vi "Processing the state after actuator action.vi"(8 "error in (no error)":errorcluster, 9 "Time to wait":i32=999, 10 "Actuator Name":string, 11 "UTP IO Session in":T1) -> (0 "error out":errorcluster, 1 "Error Text":string, 2 "Error code":i16, 3 "UTP IO Session out":T1, 4 "Result":i16, 5 "Error ocured?":bool, 7 "ExpiredTimeToWait?":bool)   [LabVIEW 2023, in "Actuators.lvlib"]
doc: "Processing the state after actuator action\nPeriod for reading is 10ms"
uses:
  Actuators.lvlib
  <vilib>/Noffz/UTP IO/UTP IO Library/Typedefs/Session Handle.ctl
  <vilib>/Noffz/UTP IO/UTP IO Library/UTP IO Pool Session.lvclass
  <vilib>/Noffz/UTP IO/UTP IO Library/methods/poly/plc/Read PLC Variable (Boolean).vi
  <vilib>/Noffz/UTP IO/UTP IO Library/methods/poly/plc/Read PLC Variable (I16).vi
  <vilib>/Noffz/UTP IO/UTP IO Library/methods/poly/plc/Read PLC Variable (String).vi
  <vilib>/Noffz/UTP IO/UTP IO Library/methods/poly/plc/Write PLC Variable (Boolean).vi
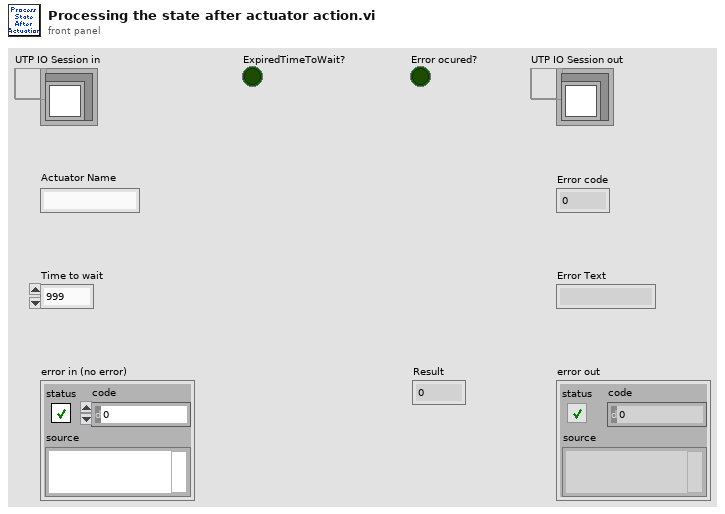
[diagram p1: front panel]
types:
  T1 = typedef "UTP IO Library.lvlib/UTP IO Pool Session.lvclass/Session Handle.ctl" = refnum<data-value>
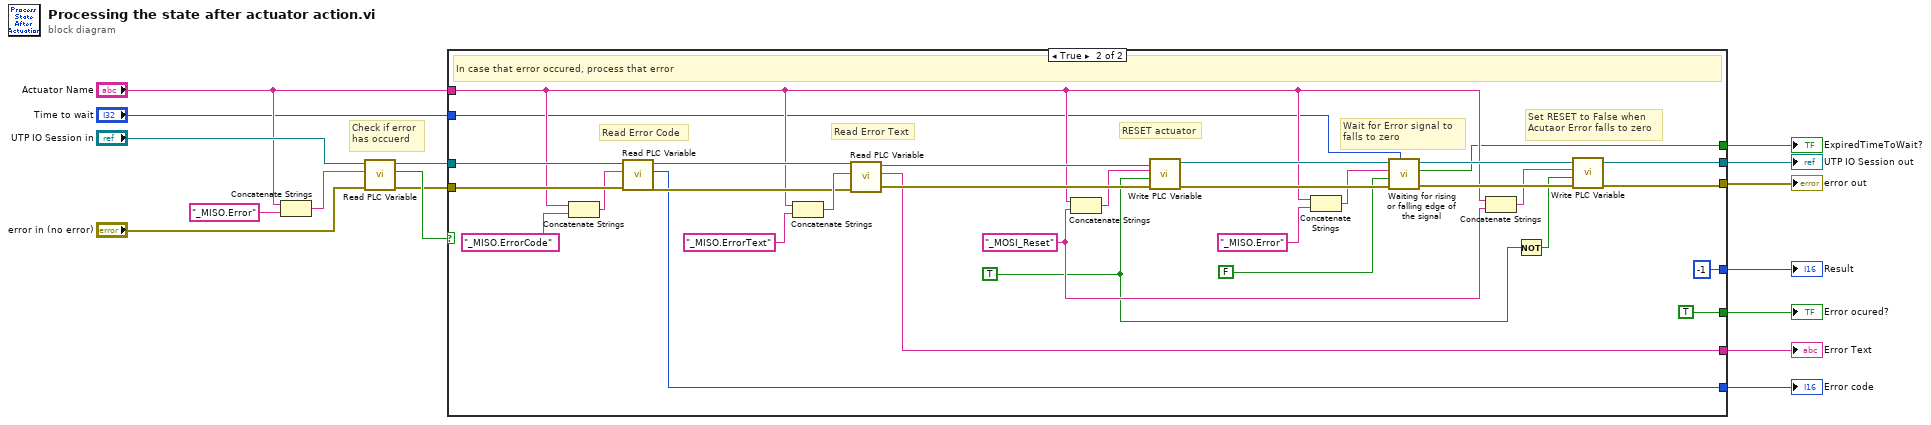
[diagram p0: block diagram]
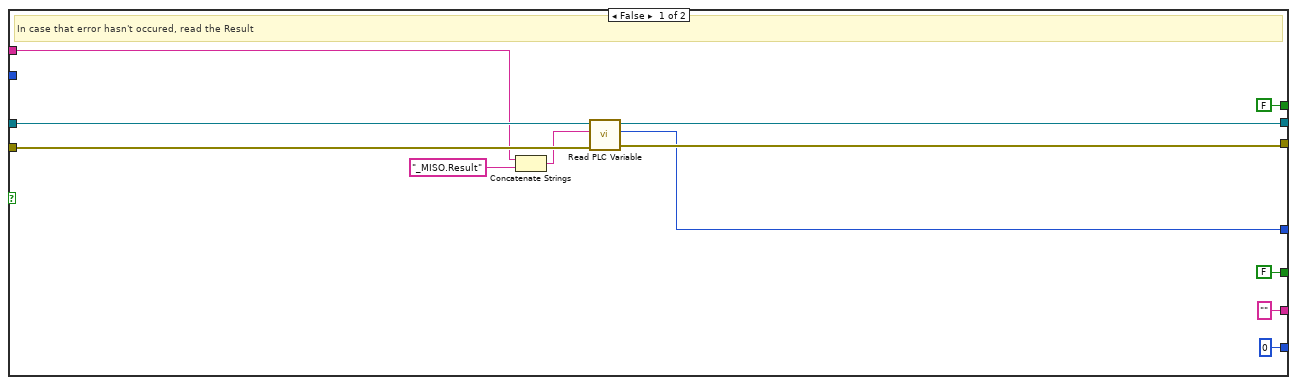
[diagram p2: hidden frame]
diagram:
  # "Check if error\nhas occuerd"
  n1 = Concatenate Strings("Actuator Name", "_MISO.Error" ("string")) -> (w14:string)
  n2 = call-poly <vilib>:"Read PLC Variable.vi"("error in (no error)"="error in (no error)", "variable name"=w14, "UTP IO Session in"="UTP IO Session in") -> ("error out"=w10:errorcluster, "value"=w15:bool, "UTP IO Session out"=w11:T1)  [unwired: 6 in]
  n3 = case shown="True" w15 {
    tunnel: w11 -> [w25 w59]
    tunnel: w10 -> [w23 w58]
    tunnel: "Actuator Name" -> [w19 w33]
    tunnel: [w24 w39] -> w3
    tunnel: [w22 w38] -> w8
    tunnel: ["" ("value") w37] -> w7
    tunnel: [i16 0 ("value") w36] -> w6
    tunnel: [FALSE ("Rising/Falling edge") TRUE ("Rising/Falling edge")] -> w5
    tunnel: [w18 i16 -1 ("value")] -> w4
    tunnel: [FALSE ("Expired3s?") w30] -> w2
    tunnel: "Time to wait" -> [_ w29]
    frame False {
      # "In case that error hasn't occured, read the Result"
      n4 = Concatenate Strings(w19, "_MISO.Result" ("string")) -> (w21:string)
      n5 = call-poly <vilib>:"Read PLC Variable.vi"("error in (no error)"=w23, "variable name"=w21, "UTP IO Session in"=w25) -> ("error out"=w22:errorcluster, "value"=w18:i16, "UTP IO Session out"=w24:T1)  [unwired: 6 in]
    }
    frame True {
      w40 = TRUE ("value")
      w43 = "_MOSI_Reset" ("string")
      # "Set RESET to False when\nAcutaor Error falls to zero"
      # "Wait for Error signal to \nfalls to zero"
      # "RESET actuator"
      # "Read Error Text"
      # "Read Error Code"
      # "In case that error occured, process that error"
      n6 = Concatenate Strings(w33, "_MISO.ErrorCode" ("string")) -> (w57:string)
      n7 = call-poly <vilib>:"Read PLC Variable.vi"("error in (no error)"=w58, "variable name"=w57, "UTP IO Session in"=w59) -> ("error out"=w52:errorcluster, "value"=w36:i16, "UTP IO Session out"=w56:T1)  [unwired: 6 in]
      n8 = Concatenate Strings(w33, "_MISO.ErrorText" ("string")) -> (w53:string)
      n9 = call-poly <vilib>:"Read PLC Variable.vi"("error in (no error)"=w52, "variable name"=w53, "UTP IO Session in"=w56) -> ("error out"=w50:errorcluster, "value"=w37:string, "UTP IO Session out"=w51:T1)  [unwired: 6 in]
      n10 = Concatenate Strings(w33, w43) -> (w49:string)
      n11 = call-poly <vilib>:"Write PLC Variable.vi"("error in (no error)"=w50, "value"=w40, "variable name"=w49, "UTP IO Session in"=w51) -> ("error out"=w47:errorcluster, "UTP IO Session out"=w48:T1)  [unwired: 6 in]
      n12 = Concatenate Strings(w33, "_MISO.Error" ("string")) -> (w31:string)
      n13 = call "Waiting for rising or falling edge of the signal.vi"("Time to wait"=w29, "error in"=w47, "Rising/Falling edge"=FALSE, "Variable name"=w31, "UTP IO Session in"=w48) -> ("error out"=w44:errorcluster, "ExpiredTimeToWait?"=w30:bool, "UTP IO Session out"=w45:T1)  [unwired: 4 in]
      n14 = Concatenate Strings(w33, w43) -> (w42:string)
      n15 = Not(x=w40) -> (.not. x?=w41:bool)
      n16 = call-poly <vilib>:"Write PLC Variable.vi"("error in (no error)"=w44, "value"=w41, "variable name"=w42, "UTP IO Session in"=w45) -> ("error out"=w38:errorcluster, "UTP IO Session out"=w39:T1)  [unwired: 6 in]
    }
  }
  "error out" <- w8
  "Error Text" <- w7
  "Error code" <- w6
  "Error ocured?" <- w5
  "Result" <- w4
  "UTP IO Session out" <- w3
  "ExpiredTimeToWait?" <- w2
